vi "Command Loop.vi"(8 "Error in":errorcluster, 10 "Queue Refs":variant, 11 "Device Reference in":T1 format="%.0x") -> ()   [LabVIEW 2026, in "Runtime Configuration Support Example Engine.lvlib"]
uses:
  Runtime Configuration Support Example Engine.lvlib
  <vilib>/NI VeriStand/Custom Device API/Custom Device Item Ref.ctl
  <vilib>/NI VeriStand/Custom Device API/Message Response (String).ctl
  <vilib>/NI VeriStand/Custom Device API/Message Response (Byte Array).ctl
  <vilib>/NI VeriStand/Custom Device API/Custom Device API.lvlib
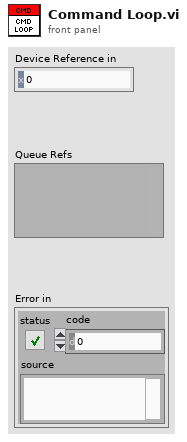
[diagram p1: front panel]
types:
  T1 = typedef "Custom Device API.lvlib/Custom Device Item Ref.ctl" = u64
  T2 = typedef "Custom Device API.lvlib/Custom Device Engine Event Ref.ctl" = refnum<event-registration>
  T3 = typedef "Custom Device API.lvlib/Message Response (String).ctl" = cluster{"Response":string, "Error":errorcluster}
  T4 = typedef "Custom Device API.lvlib/Message Response (Byte Array).ctl" = cluster{"Response":u8[], "Error":errorcluster}
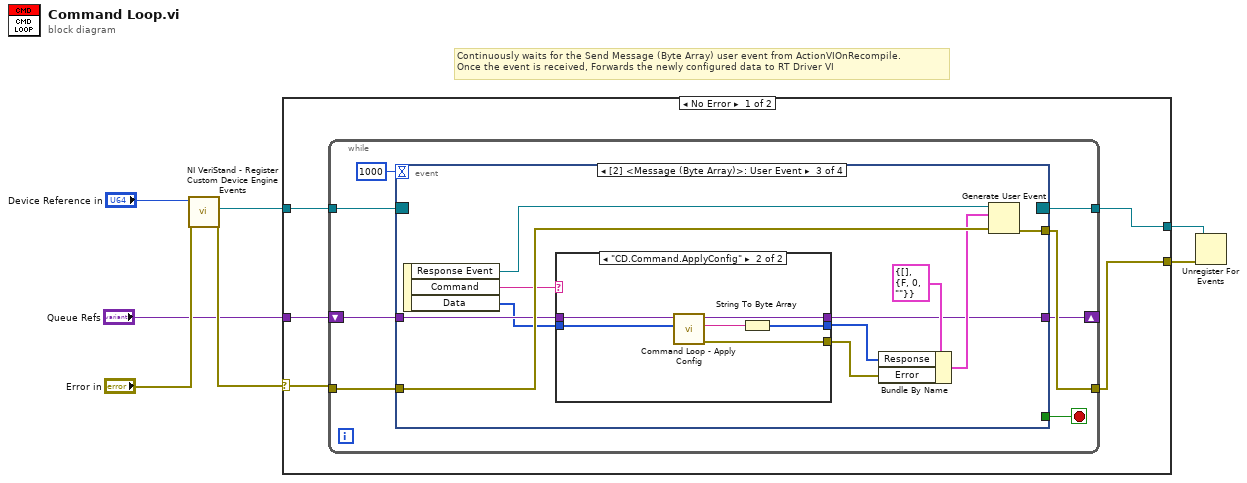
[diagram p0: block diagram]
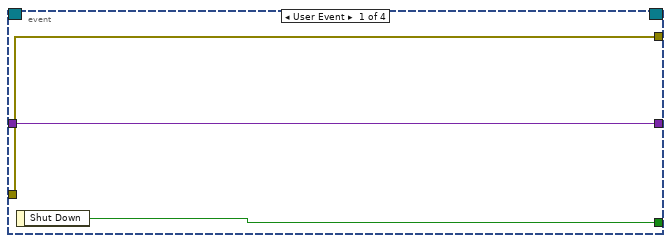
[diagram p2: hidden frame]
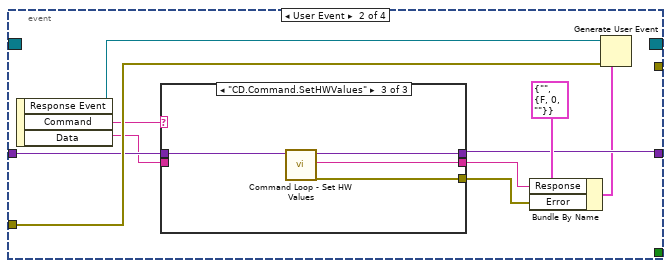
[diagram p3: hidden frame]
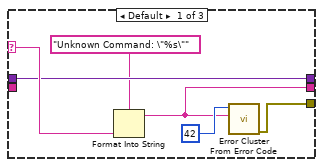
[diagram p4: hidden frame]
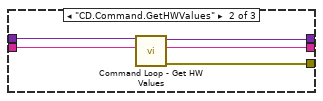
[diagram p5: hidden frame]
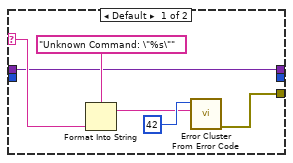
[diagram p6: hidden frame]
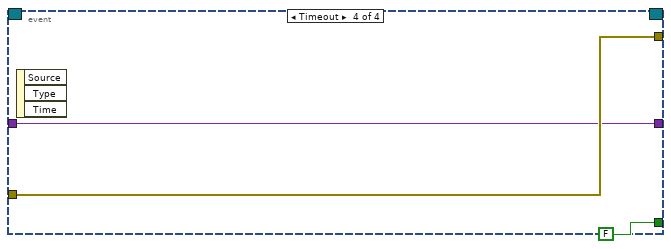
[diagram p7: hidden frame]
diagram:
  # "Continuously waits for the Send Message (Byte Array) user event from ActionVIOnRecompile.\nOnce the event is received, Forwards the newly configured data to RT Driver VI"
  n1 = call <vilib>:"NI VeriStand - Register Custom Device Engine Events.vi"("error in (no error)"="Error in", "Device Ref in"="Device Reference in") -> ("error out"=w5:errorcluster, "Custom Device Engine Event Ref"=w2:T2)  [unwired: 7 in, 1 out]
  n2 = case shown="No Error" w5 {
    selector: w5 -> [w12 w75]
    tunnel: [w10 _] -> w4
    tunnel: [w11 w75] -> w7
    tunnel: w2 -> [w9 _]
    tunnel: "Queue Refs" -> [w8 _]
    frame No Error {
      n3 = while {
        tunnel: [w17] -> w10
        tunnel: w9 -> [w16]
        shift-right: [w13] -> _
        shift-left: w8 -> [w14]
        tunnel: w12 -> [w20]
        tunnel: [w19] -> w11
        stop <- w18 stop-if-true
        n4 = event shown="[2] <Message (Byte Array)>: User Event" {
          selector: w16 -> [_ _ _ _]
          dyn-events: [_ _ _ _] -> w17
          timeout: 1000 -> [_ _ _ _]
          tunnel: [w22 _ _ FALSE ("Shut Down")] -> w18
          tunnel: [w23 _ w57 w74] -> w19
          tunnel: w20 -> [w23 w33 w58 w74]
          tunnel: w14 -> [w21 w28 w51 w72]
          tunnel: [w21 w27 w50 w72] -> w13
          event User Event {
            n5 = event-data() -> ("Shut Down"=w22:bool)  [unwired: 1 in]
          }
          event User Event {
            n6 = event-data() -> ("Response Event"=w29:refnum<user-event>, "Command"=w30:string, "Data"=w26:string)  [unwired: 1 in]
            n7 = case shown="\"CD.Command.SetHWValues\"" w30 {
              selector: w30 -> [w37 _ _]
              tunnel: w28 -> [w36 w43 w47]
              tunnel: [w36 w40 w46] -> w27
              tunnel: w26 -> [_ w42 _]
              tunnel: [w34 w41 w45] -> w24
              tunnel: [w39 w44 w48] -> w32
              frame Default {
                n8 = Format Into String(format string="Unknown Command: \"%s\"", w37) -> (resulting string=w34:string)  [unwired: 2 in, 1 out]
                n9 = call <vilib>:"Error Cluster From Error Code.vi"("error message (\"\")"=w34, "error code (0)"=42) -> ("error out"=w39:errorcluster)  [unwired: 7 in]
              }
              frame "CD.Command.GetHWValues" {
                n10 = call "Command Loop - Get HW Values.vi"("Data"=w42, "Queue Refs in"=w43) -> ("error out"=w44:errorcluster, "Response"=w41:string, "Queue Refs out"=w40:variant)  [unwired: 7 in]
              }
              frame "CD.Command.SetHWValues" {
                n11 = call "Command Loop - Set HW Values.vi"("Queue Refs in"=w47) -> ("error out"=w48:errorcluster, "Response"=w45:string, "Queue Refs out"=w46:variant)  [unwired: 8 in]
              }
            }
            n12 = Bundle By Name(cluster=T3 {"Response"="", "Error"={"status"=FALSE, "code"=0, "source"=""}} ("event data"), "Response"=w24, "Error"=w32) -> (w25:T3)
            n13 = Generate User Event(user event=w29, event data cluster=w25, error in=w33) -> ()  [unwired: 1 in, 2 out]
          }
          event User Event {
            n14 = event-data() -> ("Response Event"=w56:refnum<user-event>, "Command"=w52:string, "Data"=w49:u8[])  [unwired: 1 in]
            n15 = case shown="\"CD.Command.ApplyConfig\"" w52 {
              selector: w52 -> [w62 _]
              tunnel: [w65 w71] -> w59
              tunnel: [_ w66] -> w54
              tunnel: w51 -> [w60 w70]
              tunnel: [w60 w69] -> w50
              tunnel: w49 -> [_ w68]
              frame Default {
                n16 = Format Into String(format string="Unknown Command: \"%s\"", w62) -> (resulting string=w61:string)  [unwired: 2 in, 1 out]
                n17 = call <vilib>:"Error Cluster From Error Code.vi"("error message (\"\")"=w61, "error code (0)"=42) -> ("error out"=w65:errorcluster)  [unwired: 7 in]
              }
              frame "CD.Command.ApplyConfig" {
                n18 = call "Command Loop - Apply Config.vi"("Data"=w68, "Queue Refs in"=w70) -> ("error out"=w71:errorcluster, "Response"=w67:string, "Queue Refs out"=w69:variant)  [unwired: 7 in]
                n19 = String To Byte Array(string=w67) -> (unsigned byte array=w66:u8[])
              }
            }
            n20 = Bundle By Name(cluster=T4 {"Response"=[], "Error"={"status"=FALSE, "code"=0, "source"=""}} ("event data"), "Response"=w54, "Error"=w59) -> (w53:T4)
            n21 = Generate User Event(user event=w56, event data cluster=w53, error in=w58) -> (error out=w57:errorcluster)  [unwired: 1 in, 1 out]
          }
          event Timeout {
            n22 = event-data() -> ()  [unwired: 1 in, 3 out]
          }
        }
      }
    }
    frame Error {
    }
  }
  n23 = Unregister For Events(event registration refnum=w4, error in=w7) -> ()  [unwired: 1 out]
